vi "Approach_withSR570_over_RS232.vi"(7 "Computer called (T/F)":bool) -> ()   [LabVIEW 2023]
uses:
  Settings.vi
  Sub_Vi/TypeDefs/WayPointCluster.ctl
  Sub_Vi/TypeDefs/Settings.ctl
  Sub_Vi/TypeDefs/ChangeOnFly.ctl
  Sub_Vi/TypeDefs/Display.ctl
  Sub_Vi/TypeDefsControls/Zposition.ctl
  Sub_Vi/TypeDefsControls/Piezo Velocity.ctl
  Sub_Vi/TypeDefsControls/Voltage.ctl
  Sub_Vi/TypeDefsControls/Feedback Type.ctl
  Sub_Vi/TypeDefsControls/Xposition.ctl
  Sub_Vi/TypeDefsControls/Yposition.ctl
panel:
  in  "VISA resource name":refnum<visa-resource-name>
  in  "Filter Type (5:none)":u16(ring)=5 items=["6 dB highpass", "12 dB highpass", "6 dB bandpass", "6 dB lowpass", "12 dB lowpass", "none"]
  in  "Low Frequency Half Power Point (0: 0.03 Hz)":u16(ring) items=["0.03 Hz", "0.1 Hz", "0.3 Hz", "1 Hz", "3 Hz", "10 Hz", "30 Hz", "100 Hz", "300 Hz", "1 kHz", "3 kHz", "10 kHz", "30 kHz", "100 kHz", "300 kHz", "1 MHz"]
  in  "High Frequency Half Power Point (0: 0.03 Hz)":u16(ring) items=["0.03 Hz", "0.1 Hz", "0.3 Hz", "1 Hz", "3 Hz", "10 Hz", "30 Hz", "100 Hz", "300 Hz", "1 kHz", "3 kHz", "10 kHz"]
  in  "Sensitivity (0:1 pA/V)":u16(ring) items=["1 pA/V", "2 pA/V", "5 pA/V", "10 pA/V", "20 pA/V", "50 pA/V", "100 pA/V", "200 pA/V", "500 pA/V", "1 nA/V", "2 nA/V", "5 nA/V", "10 nA/V", "20 nA/V", "50 nA/V", "100 nA/V", "200 nA/V", "500 nA/V", "1 µA/V", "2 µA/V", "5 µA/V", "10 µA/V", "20 µA/V", "50 µA/V", "100 µA/V", "200 µA/V", "500 µA/V", "1 mA/V"]
  in  "Gain Mode (0: Low Noise)":u16(ring) items=["Low Noise", "High Bandwidth", "Low Drift"]
  in  "Bias Voltage Level (0.000 V)":i32
  out "Current 5":cluster{"Y":dbl[], "Y":dbl[]}[](graph)
  out "Current 4":cluster{"Y":dbl[], "Y":dbl[]}[](graph)
  out "Lock In Phase":dbl[](graph)
  out "Lock In Amplitude":dbl[](graph)
  in  "Start scan Button":bool
  in  "Retract after approach over":bool=TRUE
  in  "Display Cluster":T1
  in  "ChangeonFly":T2
  in  "SettingsCluster":T3={"Sample Rate (us)"=1, "Samples Per Data Point (int, power of 2)"=1000, "DistanceToBulk (um)"=-1.0, "HoldTimeScaler"=1, "SaveData"=TRUE, "DistanceToBulk (um) 2"=-1.0, "DistanceToBulk (um) 3"=-1.0}
  in  "WayPointCluster":T4
  in  "Feedback Type":T5
  in  "Tab Control":enum32{"Current-Distance", "Current-Time"}(tab)
  out "Current 1":cluster{"Y":dbl[], "Y":dbl[]}[](graph)
  out "Current 2":cluster{"Y":dbl[], "Y":dbl[]}[](graph)
  out "Current 3":cluster{"Y":dbl[], "Y":dbl[]}[](graph)
  out "Current 1":dbl[](graph)
  out "Current 2":dbl[](graph)
  out "Current 3":dbl[](graph)
  in  "Feedback Threshold (A)":dbl=1e-13 min=-360.0 max=360.0
  in  "Greater Than":bool=TRUE
  in  "Set X":bool
  in  "Set Y":bool
  in  "Y (µm)":T6=50.0 min=0.0 max=100000.0
  in  "X (µm)":T7=50.0 min=0.0 max=100000.0
  in  "Approach Voltage (V)":T8=0.35 min=-10.0 max=10.0
  in  "Approach Rate (µm/s)":T9=0.1 min=0.0
  in  "End Extension (µm)":T10=38.0 min=0.0 max=100000.0
  in  "Start Extention (µm)":T10 min=0.0 max=100000.0
  in  "stop 2":bool
  in  "Pause":bool
  # "Settings"
  # "SR570 Settings"
  # "Pause at"
  # "Advanced Settings"
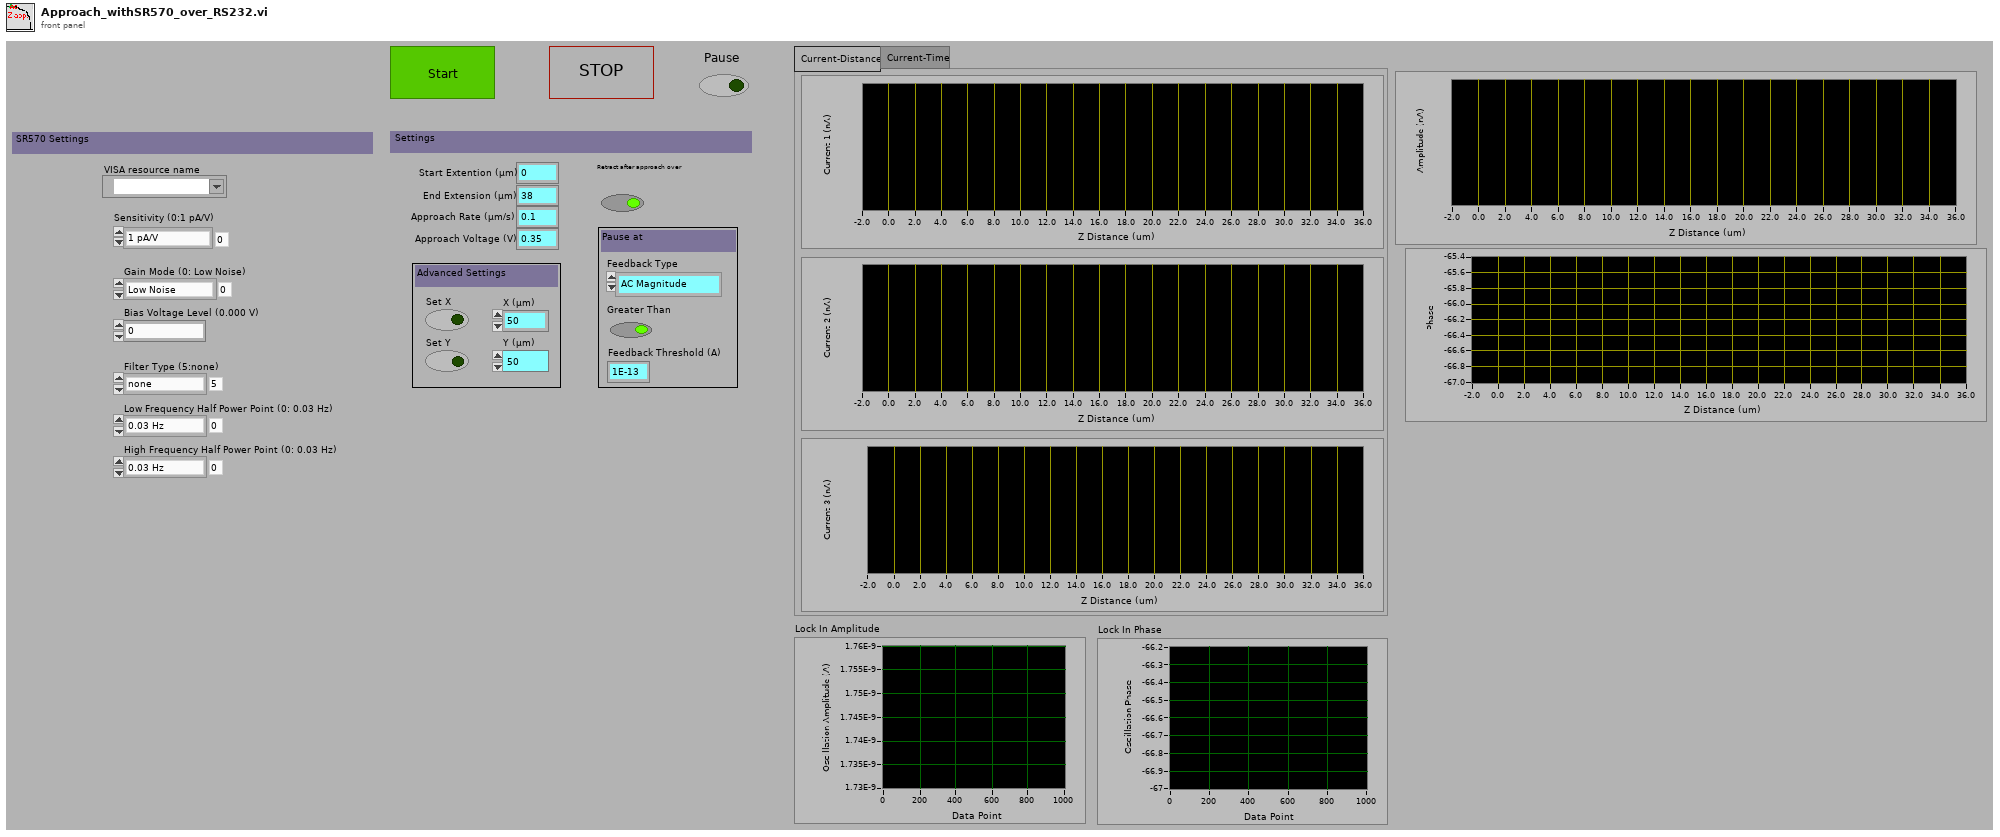
[diagram p1: front panel]
types:
  T1 = typedef "Display.ctl" = cluster{"X":refnum<vi>, "Y":refnum<vi>, "Z":refnum<vi>, "Amp":refnum<vi>, "Phase":refnum<vi>, "t vs Z":refnum<vi>, "t vs C1":refnum<vi>, "t vs C2":refnum<vi>, "t vs C3":refnum<vi>, "t vs Amp":refnum<vi>, "t vs Phase":refnum<vi>, "t vs X":refnum<vi>, "t vs Y":refnum<vi>, "Z vs C1":refnum<vi>, "Z vs C2":refnum<vi>, "Z vs C3":refnum<vi>, "V vs C1":refnum<vi>, "V vs C2":refnum<vi>, "V vs C3":refnum<vi>, "X/Y/Z F":refnum<vi>, "X/Y/Z R":refnum<vi>, "X/Y/C1 F":refnum<vi>, "X/Y/C1 R":refnum<vi>, "X/Y/C2 F":refnum<vi>, "X/Y/C2 R":refnum<vi>, "X/Y/C3 F":refnum<vi>, "X/Y/C3 R":refnum<vi>, "NumberOfLines":u16, "um Per Pixel":dbl, "um Per Line":dbl, "X Center":dbl, "Hop X/Y/Z":refnum<vi>, "Hop X/Y/C1":refnum<vi>, "Hop X/Y/C2":refnum<vi>, "Hop X/Y/C3":refnum<vi>, "X Width":dbl, "Y Width":dbl, "Hopping Distance":dbl, "V2 vs C1":refnum<vi>, "V vs Phase":refnum<vi>, "Y Center":dbl, "Number of Pixels":dbl, "V2 vs C2":refnum<vi>, "V2 vs C3":refnum<vi>, "V vs y":refnum<vi>, "V2 vs y":refnum<vi>, "Z vs Amp":refnum<vi>, "Z vs Phase":refnum<vi>}
  T2 = typedef "ChangeOnFly.ctl" = cluster{"Stop (boolean)":refnum<vi>, "Pause (boolean)":refnum<vi>, "EndCurrentLine (boolean)":refnum<vi>, "max movement per update step (Interger, nm)":refnum<vi>, "P (float, arb)":refnum<vi>, "Feedback set point (double, Amps)":refnum<vi>, "Voltage (double, V)":refnum<vi>, "Feedback set point 2 (double, Amps)":refnum<vi>, "Stop on Greater Than 2? (boolean)":refnum<vi>, "Stop on Greater Than? (boolean)":refnum<vi>, "Voltage 2 (double, V)":refnum<vi>, "Feedback Type (enum)":refnum<vi>, "Feedback Type 2 (enum)":refnum<vi>}
  T3 = typedef "Settings.ctl" = cluster{"Sample Rate (us)":u32, "Samples Per Data Point (int, power of 2)":i16, "DistanceToBulk (um)":dbl, "HoldTimeScaler":u64, "SaveData":bool, "DistanceToBulk (um) 2":dbl, "DistanceToBulk (um) 3":dbl}
  T4 = typedef "WayPointCluster.ctl" = cluster{"X (um)":dbl[], "Y (um)":dbl[], "Z (um)":dbl[], "V (V)":dbl[], "X Velocity (um s-1)":dbl[], "Y Velocity (um s-1)":dbl[], "Z Velocity (um s-1)":dbl[], "V Velocity (V s-1)":dbl[], "FeedBack Type (enum)":u16[], "Move X (boolean)":bool[], "Move Y (boolean)":bool[], "Move Z (boolean)":bool[], "Move V (boolean)":bool[], "Jump V (boolean)":bool[], "Hold (boolean)":bool[], "Hold Time":u32[], "V2 (V)":dbl[], "Move V2":bool[], "V2 Velocity (V s-1)":dbl[], "Jump V2 (boolean)":bool[], "Update z Position delta (ms)":i16[], "Hold Feedback1":bool[], "Move Z PicoMotor":bool[], " Z PicoMotor Direction":bool[], "DIO0":bool[]}
  T5 = typedef "Feedback Type.ctl" = enum16{"AC Magnitude", "Current 1", "Current 2", "Phase"}
  T6 = typedef "Yposition.ctl" = dbl
  T7 = typedef "Xposition.ctl" = dbl
  T8 = typedef "Voltage.ctl" = dbl
  T9 = typedef "Piezo Velocity.ctl" = dbl
  T10 = typedef "Zposition.ctl" = dbl
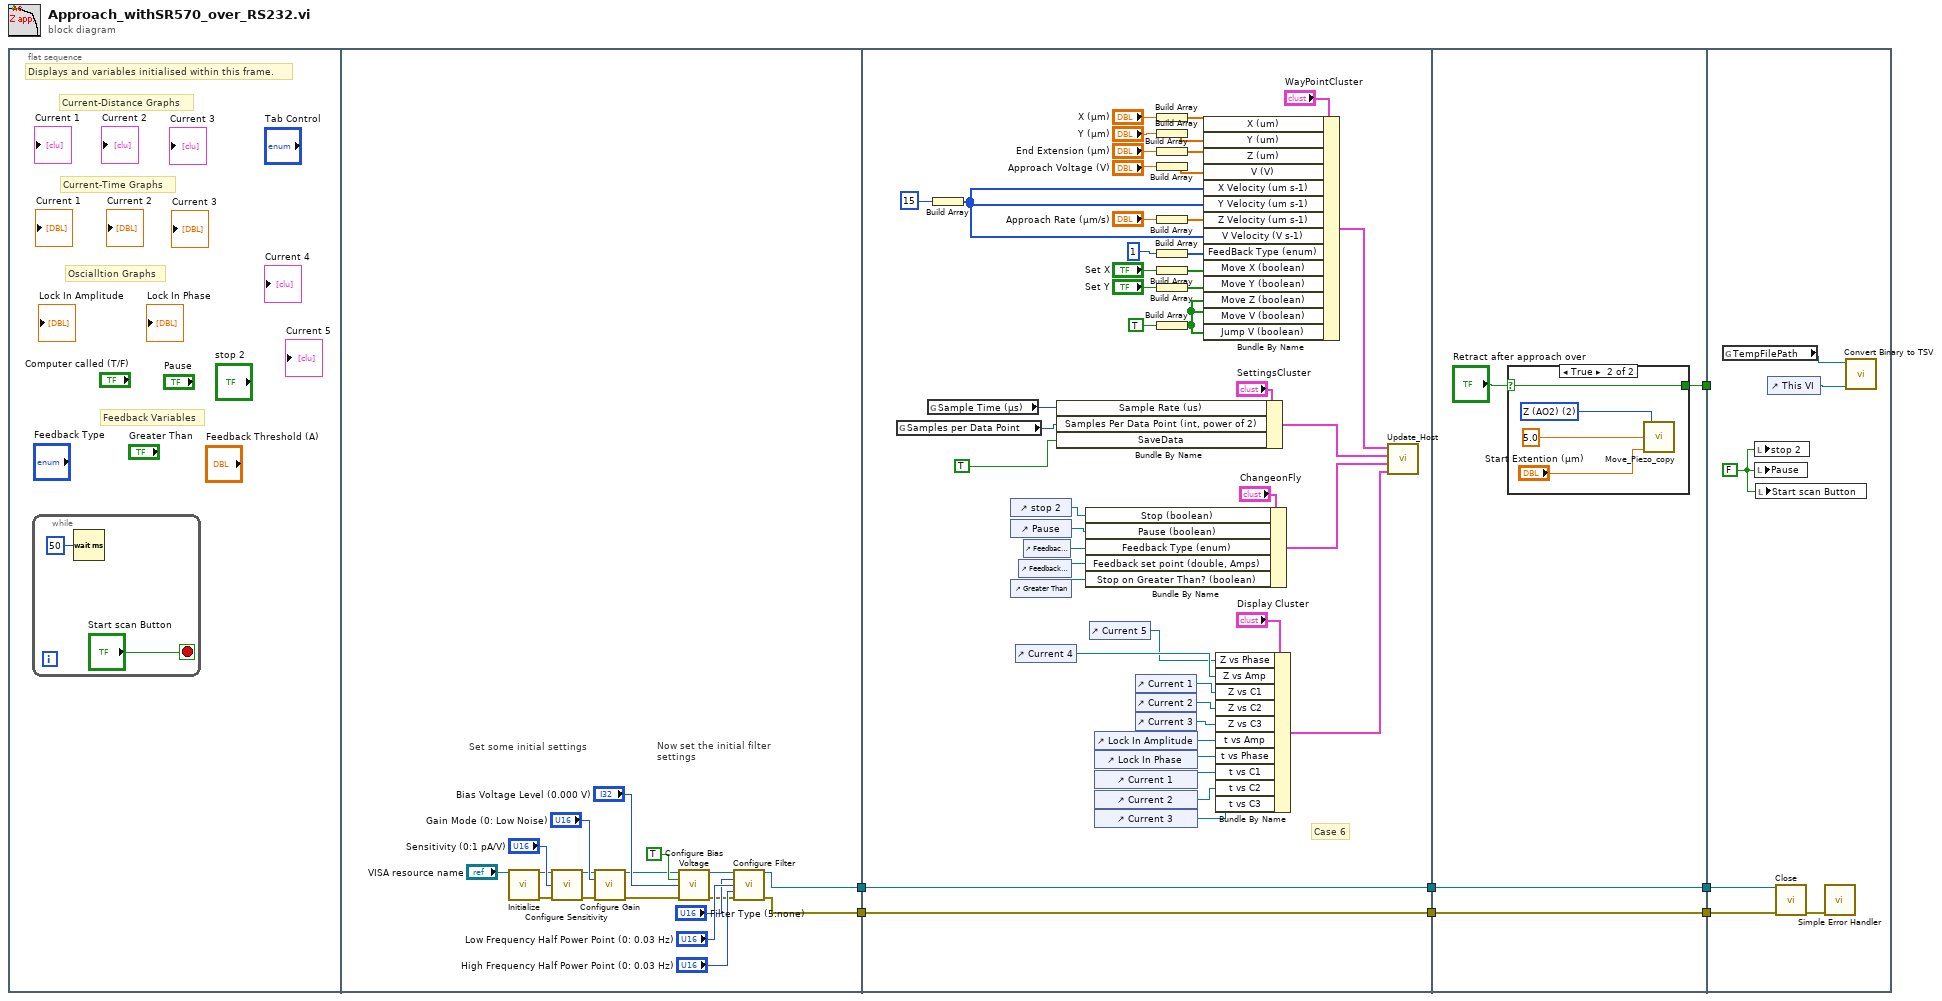
[diagram p0: block diagram]
diagram:
  n1 = flat-sequence {
    tunnel: [w11] -> w4
    tunnel: [w10] -> w1
    tunnel: [w29] -> w5
    tunnel: w4 -> [w29]
    tunnel: [w28] -> w2
    tunnel: w1 -> [w28]
    tunnel: [w78] -> w7
    tunnel: [w77] -> w6
    tunnel: w5 -> [w77]
    tunnel: [w76] -> w3
    tunnel: w2 -> [w76]
    tunnel: w7 -> [_]
    tunnel: w6 -> [w86]
    tunnel: w3 -> [w85]
    frame #0 {
      # "Feedback Variables"
      # "Oscialltion Graphs"
      # "Current-Time Graphs"
      # "Current-Distance Graphs"
      # "Displays and variables initialised within this frame."
      n2 = while {
        stop <- "Start scan Button" stop-if-true
        n3 = Wait (ms)(milliseconds to wait=u32 50) -> ()  [unwired: 1 out]
      }
    }
    frame #1 {
      # "Now set the initial filter\nsettings"
      # "Set some initial settings"
      n4 = call <instrlib>:"Initialize.vi"("VISA resource name"="VISA resource name") -> ("VISA resource name out"=w13:refnum<visa-resource-name>, "error out"=w14:errorcluster)  [unwired: 13 in]
      n5 = call <instrlib>:"Configure Sensitivity.vi"("VISA resource name"=w13, "Sensitivity (0:1 pA/V)"="Sensitivity (0:1 pA/V)", "error in (no error)"=w14) -> ("VISA resource name out"=w16:refnum<visa-resource-name>, "error out"=w17:errorcluster)  [unwired: 11 in]
      n6 = call <instrlib>:"Configure Gain.vi"("VISA resource name"=w16, "Gain Mode (0: Low Noise)"="Gain Mode (0: Low Noise)", "error in (no error)"=w17) -> ("VISA resource name out"=w19:refnum<visa-resource-name>, "error out"=w20:errorcluster)  [unwired: 11 in]
      n7 = call <instrlib>:"Configure Bias Voltage.vi"("VISA resource name"=w19, "Enable Bias Voltage (F:Disable)"=TRUE, "Bias Voltage Level (0.000 V)"="Bias Voltage Level (0.000 V)", "error in (no error)"=w20) -> ("VISA resource name out"=w23:refnum<visa-resource-name>, "error out"=w24:errorcluster)  [unwired: 10 in]
      n8 = call <vilib>:"Configure Filter.vi"("VISA resource name"=w23, "Filter Type (5:none)"="Filter Type (5:none)", "Low Frequency Half Power Point (0: 0.03 Hz)"="Low Frequency Half Power Point (0: 0.03 Hz)", "High Frequency Half Power Point (0: 0.03 Hz)"="High Frequency Half Power Point (0: 0.03 Hz)", "error in (no error)"=w24) -> ("VISA resource name out"=w11:refnum<visa-resource-name>, "error out"=w10:errorcluster)  [unwired: 9 in]
    }
    frame #2 {
      # "Case 6"
      n9 = global read "Settings.vi" "Samples per Data Point"() -> (w52:u16)
      n10 = global read "Settings.vi" "Sample Time (µs)"() -> (w53:u32)
      n11 = Build Array(15) -> (w75:i32[])
      n12 = control-ref of="stop 2"() -> (w45:refnum<vi>)
      n13 = control-ref of="Pause"() -> (w64:refnum<vi>)
      n14 = control-ref of="Greater Than"() -> (w50:refnum<vi>)
      n15 = control-ref of="Current 4"() -> (w32:refnum<vi>)
      n16 = control-ref of="Feedback Threshold (A)"() -> (w65:refnum<vi>)
      n17 = control-ref of="Feedback Type"() -> (w49:refnum<vi>)
      n18 = Bundle By Name(cluster="SettingsCluster", "Sample Rate (us)"=w53, "Samples Per Data Point (int, power of 2)"=w52, "SaveData"=TRUE) -> (w35:T3)
      n19 = Bundle By Name(cluster="ChangeonFly", "Stop (boolean)"=w45, "Pause (boolean)"=w64, "Feedback Type (enum)"=w49, "Feedback set point (double, Amps)"=w65, "Stop on Greater Than? (boolean)"=w50) -> (w34:T2)
      n20 = control-ref of="Current 5"() -> (w31:refnum<vi>)
      n21 = control-ref of="Lock In Amplitude"() -> (w33:refnum<vi>)
      n22 = control-ref of="Lock In Phase"() -> (w62:refnum<vi>)
      n23 = control-ref of="Current 1"() -> (w42:refnum<vi>)
      n24 = control-ref of="Current 2"() -> (w46:refnum<vi>)
      n25 = control-ref of="Current 3"() -> (w61:refnum<vi>)
      n26 = control-ref of="Current 1"() -> (w69:refnum<vi>)
      n27 = control-ref of="Current 2"() -> (w43:refnum<vi>)
      n28 = control-ref of="Current 3"() -> (w44:refnum<vi>)
      n29 = Build Array("X (µm)") -> (w74:T7[])
      n30 = Build Array("Y (µm)") -> (w73:T6[])
      n31 = Build Array("End Extension (µm)") -> (w71:T10[])
      n32 = Build Array("Approach Voltage (V)") -> (w72:T8[])
      n33 = Build Array("Approach Rate (µm/s)") -> (w70:T9[])
      n34 = Build Array(u16 1) -> (w68:u16[])
      n35 = Build Array("Set X") -> (w67:bool[])
      n36 = Build Array("Set Y") -> (w66:bool[])
      n37 = Build Array(TRUE ("Save Data")) -> (w48:bool[])
      n38 = Bundle By Name(cluster="WayPointCluster", "X (um)"=w74, "Y (um)"=w73, "Z (um)"=w71, "V (V)"=w72, "X Velocity (um s-1)"=w75, "Y Velocity (um s-1)"=w75, "Z Velocity (um s-1)"=w70, "V Velocity (V s-1)"=w75, "FeedBack Type (enum)"=w68, "Move X (boolean)"=w67, "Move Y (boolean)"=w66, "Move Z (boolean)"=w48, "Move V (boolean)"=w48, "Jump V (boolean)"=w48) -> (w36:T4)
      n39 = Bundle By Name(cluster="Display Cluster", "Z vs Phase"=w31, "Z vs Amp"=w32, "Z vs C1"=w69, "Z vs C2"=w43, "Z vs C3"=w44, "t vs Amp"=w33, "t vs Phase"=w62, "t vs C1"=w42, "t vs C2"=w46, "t vs C3"=w61) -> (w47:T1)
      n40 = call "Update_Host.vi"("Display Cluster"=w47, "ChangeonFly"=w34, "SettingsCluster"=w35, "WayPointCluster"=w36) -> ()  [unwired: 6 in]
    }
    frame #3 {
      n41 = case shown="True" "Retract after approach over" {
        selector: "Retract after approach over" -> [w80 w83]
        tunnel: [w80 w83] -> w78
        frame False {
        }
        frame True {
          w84 = u16 2 items=["X (AO0)", "Y (AO1)", "Z (AO2)", "V (AO3)", "V2 (AO4)"] ("Piezo")
          n42 = call "Move_Piezo_copy.vi"("Piezo"=w84, "Movement Speed (µm/s)"=5.0 ("Scan Rate (um/s)"), "Position (µm) (or V)"="Start Extention (µm)") -> ()  [unwired: 13 in]
        }
      }
    }
    frame #4 {
      w89 = FALSE ("stop recording")
      n43 = global read "Settings.vi" "TempFilePath"() -> (w88:path)
      n44 = local write "stop 2"(w89) -> ()
      n45 = local write "Pause"(w89) -> ()
      n46 = local write "Start scan Button"(w89) -> ()
      n47 = control-ref of="This VI"() -> (w90:refnum<vi>)
      n48 = call <instrlib>:"Close.vi"("VISA resource name"=w86, "error in (no error)"=w85) -> ("error out"=w87:errorcluster)  [unwired: 13 in]
      n49 = call <vilib>:"Simple Error Handler.vi"("error in (no error)"=w87) -> ()  [unwired: 4 in, 5 out]
      n50 = call "Convert Binary to TSV.vi"("This VI"=w90, "TDMS DataFile Name"=w88) -> ()  [unwired: 10 in]
    }
  }
